vi "IRISS_FPGA_IO_v3.3b.vi"() -> ()   [LabVIEW 2013]
doc: "This VI contains a basic quadrature decoder which is reset asynchronously upon clicking the reset button."
uses:
  <vilib>/Platform/TimedLoop/XDataNode/timing_clust.ctl
  <vilib>/Platform/TimedLoop/XDataNode/nitl_modes.ctl
  <vilib>/Platform/TimedLoop/XDataNode/wakeup.ctl
  <vilib>/rvi/Emulation/niFpgaSctlEmulationGetInTimedLoop.vi
  <vilib>/rvi/Emulation/niFpgaEmulationReportErrorSimple.vi
  <vilib>/rvi/Emulation/niFpgaGetClockAttributes.vi
  <vilib>/rvi/Emulation/niFpgaCriticalErrorInLSC.vi
  <vilib>/rvi/eio/common/nirviEmuTemplateMethod_errors.vi
  <vilib>/platform/TimedLoop/XDataNode/XDataNode.xnode
  <vilib>/eio/EIONode/EIONode.xnode
  <vilib>/Platform/TimedLoop/XDataNode/XDNodeRunTimeDep.lvlib
  Library/KevinLibraryAll/labview/KevLib01.lvlib
  Library/jmslib.lvlib
panel:
  in  "Connector2/DIO10":bool
  in  "Connector2/DIO9":bool
  in  "Connector2/DIO8":bool
  in  "Connector2/DIO7":bool
  in  "Period 1 (Ticks)":u32=1000
  in  "PWM1":fxp<+,32,0>
  in  "Period (Ticks)":u32=2000
  in  "DIR OCT Mot":bool
  in  "INHB OCT Mot":bool
  out "FAULT OCT Mot":bool
  out "Position OCT Mot":i32
  out "JumpBy2Error OCT Mot":i16
  in  "Reset OCT Mot":bool
  in  "OCT Mot DC":fxp<+,32,0>
  in  "Conn0/DIO15 Button 4":bool
  in  "Conn0/DIO12 Button 1":bool
  in  "Conn0/DIO13 Button 2":bool
  out "Home OCT z":bool
  in  "DIR Y":bool
  in  "INHB Y":bool
  out "FAULT Y":bool
  out "Position Y":i32
  out "JumpBy2Error Y":i16
  in  "Reset Y":bool
  in  "Y DC":fxp<+,32,0>
  in  "DIR X":bool
  in  "INHB X":bool
  out "FAULT X":bool
  out "Position X":i32
  out "JumpBy2Error X":i16
  in  "Reset X":bool
  in  "DIR Z":bool
  in  "INHB Z":bool
  out "FAULT Z":bool
  out "Position Z":i32
  out "JumpBy2Error Z":i16
  in  "Reset Z":bool
  in  "Z DC":fxp<+,32,0>
  in  "X DC":fxp<+,32,0>
  out "samples":i32
  out "Current Monitor":u32[](array[numeric])
  out "Raw Data Response (MSB)":bool[](array[boolean])
  out "Home L4":bool
  out "Home L1":bool
  out "Home L2":bool
  out "Home L3":bool
  in  "Positive Direction C1-4":bool
  out "JumpBy2Error C1-4":i16
  out "32 bit Position C1-4":i32
  in  "Reset C1-4":bool
  in  "Positive Direction C1-1":bool
  out "JumpBy2Error C1-1":i16
  out "32 bit Position C1-1":i32
  in  "Reset C1-1":bool
  out "32 bit Position 17":i32
  in  "Reset 17":bool
  in  "Positive Direction 17":bool
  out "JumpBy2Error 17":i16
  out "32 bit Position 16":i32
  in  "Reset 16":bool
  in  "Positive Direction 16":bool
  out "JumpBy2Error 16":i16
  out "32 bit Position 15":i32
  in  "Reset 15":bool
  in  "Positive Direction 15":bool
  out "JumpBy2Error 15":i16
  out "32 bit Position 14":i32
  in  "Reset 14":bool
  in  "Positive Direction 14":bool
  out "JumpBy2Error 14":i16
  out "32 bit Position 13":i32
  in  "Reset 13":bool
  in  "Positive Direction 13":bool
  out "JumpBy2Error 13":i16
  out "32 bit Position 12":i32
  in  "Reset 12":bool
  in  "Positive Direction 12":bool
  out "JumpBy2Error 12":i16
  out "32 bit Position 10":i32
  in  "Reset 10":bool
  in  "Positive Direction 10":bool
  out "JumpBy2Error 10":i16
  out "32 bit Position 9":i32
  in  "Reset 9":bool
  in  "Positive Direction 9":bool
  out "JumpBy2Error 9":i16
  out "JumpBy2Error 3":i16
  in  "Positive Direction 3":bool
  out "JumpBy2Error 1":i16
  in  "Positive Direction 1":bool
  out "AI":i16[](array[numeric])
  out "32 bit Position 3":i32
  in  "Reset 3":bool
  in  "AO":i16[](array[numeric])=[0, 0, 0, 0, 0, 0, 0, 0]
  out "32 bit Position 1":i32
  in  "Reset 1":bool
  # "syringe pump"
  # "Accurus Buttons"
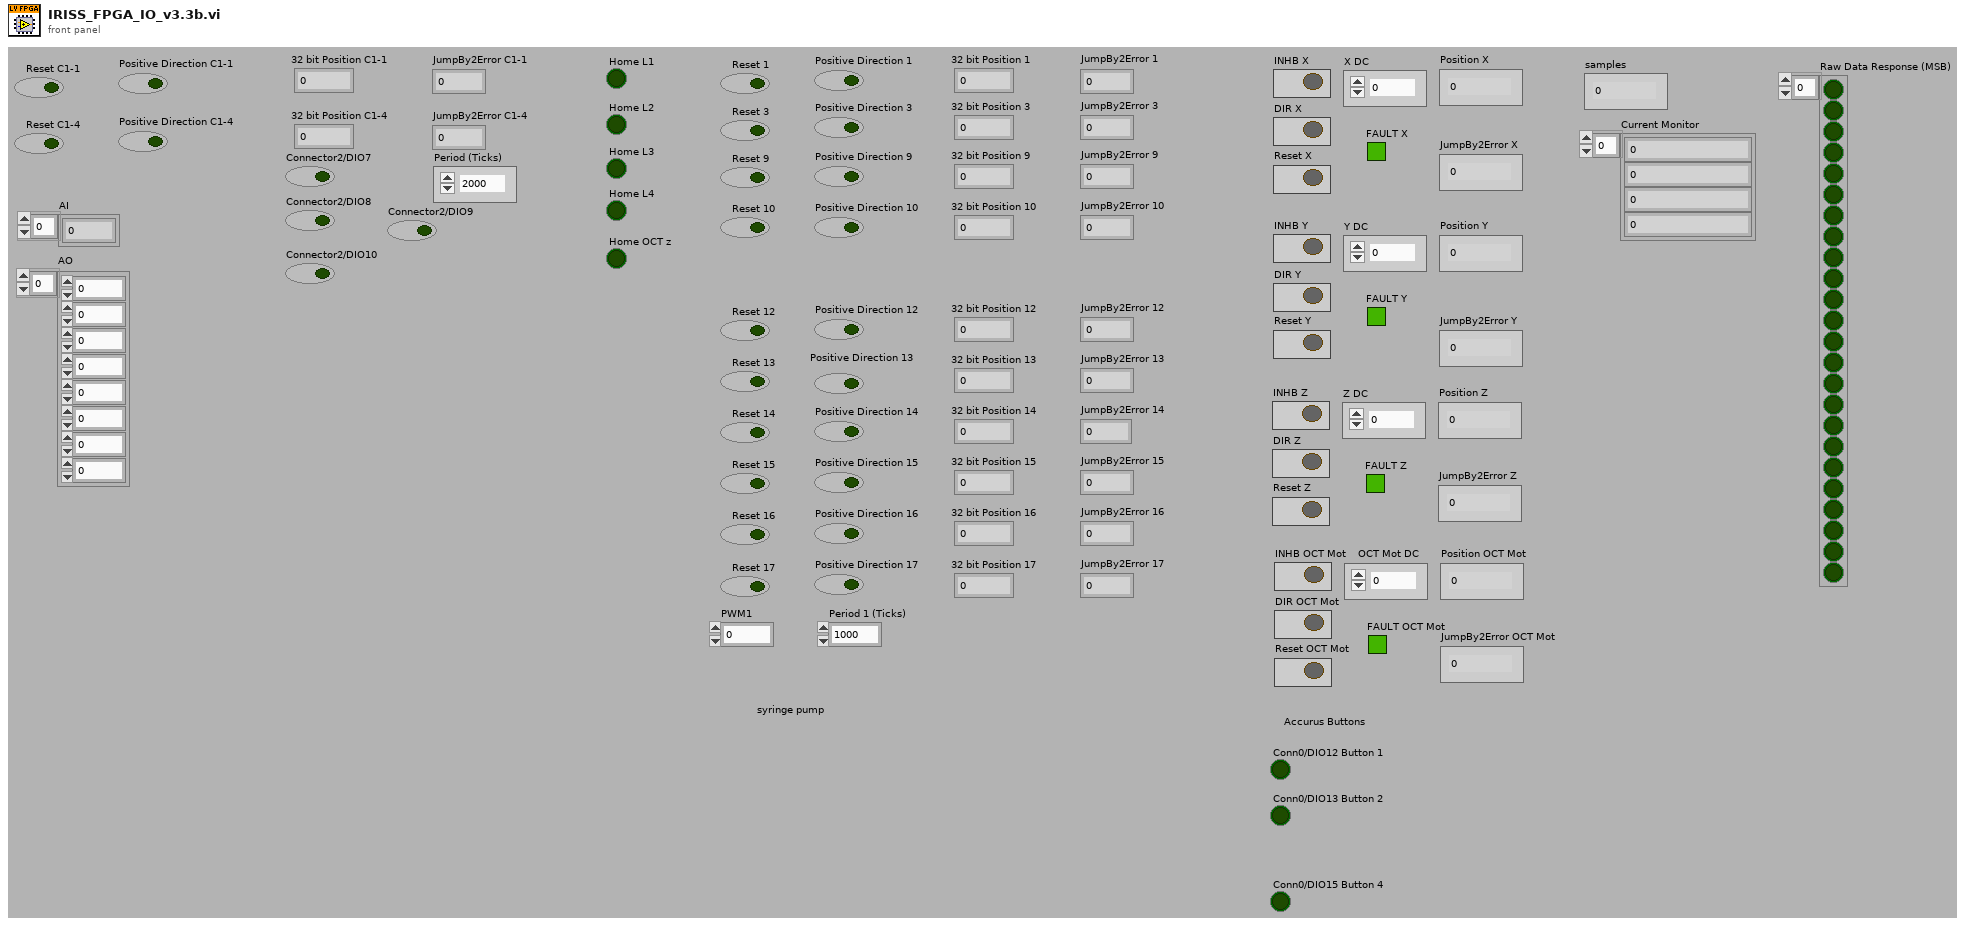
[diagram p1: front panel]
types:
  T1 = typedef "XDNodeRunTimeDep.lvlib/timing_clust.ctl" = cluster{"Expected End [f-1]":u64, "Actual End [f-1]":u64, "Finished Late? [f-1]":bool, "Expected End [i-1]":u64, "Actual End [i-1]":u64, "Finished Late? [i-1]":bool, "Expected Start [i]":u64, "Actual Start [i]":u64, "Expected Start [f]":u64, "Actual Start [f]":u64, "Source Name":string, "Structure Name":string, "Period":i64, "Deadline":i64, "Offset":i64, "Start":i64, "Priority":i32, "Timeout":i32, "Mode":T2, "Wakeup Reason":T3, "Error":errorcluster, "Source Type":string, "Secondary Source Type":string, "Global End Time":u64, "Global Start Time":u64, "Frame Duration":u64, "Iteration Duration":u64, "Assigned CPU":i32, "I/O Scan Engine Mode":u32}
  T2 = typedef "XDNodeRunTimeDep.lvlib/nitl_modes.ctl" = enum32{"No Change", "Process missed periods, maintain original phase", "Discard missed periods, maintain original phase", "Process missed periods, ignore original phase", "Discard missed periods, ignore original phase"}
  T3 = typedef "XDNodeRunTimeDep.lvlib/wakeup.ctl" = enum32{"Normal", "Aborted", "Asynchronous wakeup", "Timing source error", "Timed loop error", "Timeout"}
  T4 = cluster{"PWM In":refnum<k21>, "Direction":refnum<k21>, "Inhibit":refnum<k21>, "Encoder C":refnum<k21>, "Encoder B":refnum<k21>, "Encoder A":refnum<k21>, "Fault":refnum<k21>}
  T5 = cluster{"SCLK":refnum<k21>, "MOSI":refnum<k21>, "MISO":refnum<k21>}
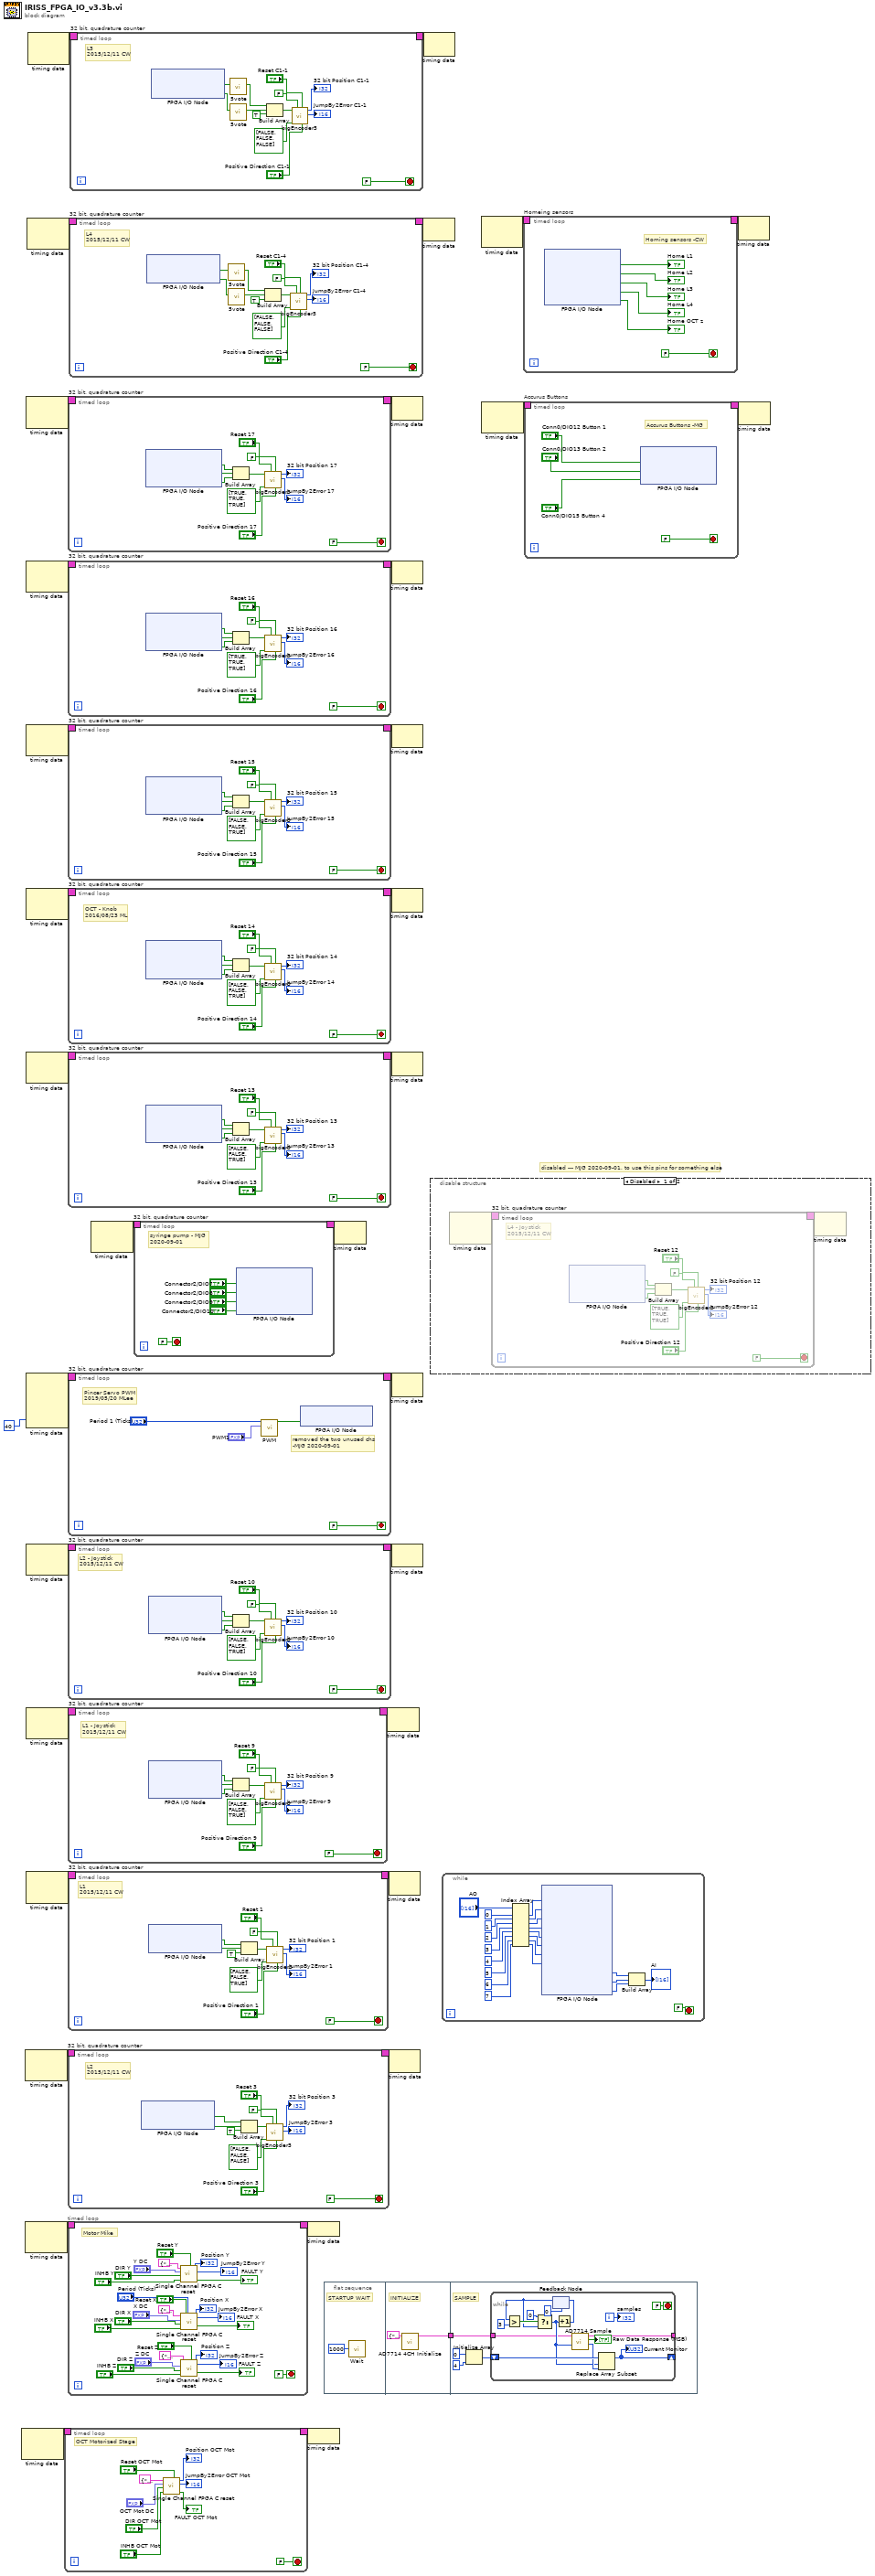
[diagram p0: block diagram]
diagram:
  # "disabled --- MJG 2020-09-01, to use this pins for something else"
  n1 = node-c288() -> (w5:T1)  [unwired: 2 in]
  n2 = node-c288() -> (w34:T1)  [unwired: 2 out]
  n3 = node-c288() -> (w10:T1)  [unwired: 2 in]
  n4 = node-c288() -> (w18:T1)  [unwired: 2 out]
  n5 = node-c288() -> (w20:T1)  [unwired: 2 out]
  n6 = node-c288() -> (w22:T1)  [unwired: 2 out]
  n7 = node-c288() -> (w24:T1)  [unwired: 2 out]
  n8 = node-c288() -> (w26:T1)  [unwired: 2 out]
  n9 = node-c288(i64 40 ("Period")) -> (w28:T1)  [unwired: 3 in, 1 out]
  n10 = node-c288() -> (w30:T1)  [unwired: 2 out]
  n11 = node-c288() -> (w32:T1)  [unwired: 2 out]
  n12 = node-c288() -> (w35:T1)  [unwired: 2 out]
  n13 = node-c288() -> (w14:T1)  [unwired: 2 out]
  n14 = node-c288() -> (w16:T1)  [unwired: 2 out]
  n15 = timed-loop {
    timing: w5 -> [_]
    timing-out: [_] -> w4
    stop <- FALSE stop-if-true
    # "OCT Motorized Stage"
    n16 = call "Single Channel FPGA C reset.vi"("Reset"="Reset OCT Mot", "INHB"="INHB OCT Mot", "DIR"="DIR OCT Mot", "Duty"="OCT Mot DC", "IO Channels"=T4 {"PWM In"="Connector1/DIO7", "Direction"="Connector1/DIO8", "Inhibit"="Connector1/DIO9", "Encoder C"="Connector1/DIO10", "Encoder B"="Connector1/DIO11", "Encoder A"="Connector1/DIO12", "Fault"="Connector1/DIO13"}) -> ("FAULT"=→"FAULT OCT Mot":bool, "JumpBy2Error"=→"JumpBy2Error OCT Mot":i16, "Position"=→"Position OCT Mot":i32)  [unwired: 4 in]
  }
  n17 = timed-loop "32 bit, quadrature counter" {
    timing-out: [_] -> w33
    timing: w34 -> [_]
    stop <- FALSE stop-if-true
    # "L2\n2015/12/11 CW"
    n18 = xnode "FPGA I/O Node"() -> ("Connector0/DIO2"=w51:bool, "Connector0/DIO3"=w50:bool)  [unwired: 2 in, 2 out]
    n19 = Build Array(w51, w50, TRUE ("element")) -> (w57:bool[])
    n20 = call "bigEncoder3.vi"("Positive Direction"="Positive Direction 3", "ForceReset"="Reset 3", "Allow C Reset?"=FALSE, "Reset Array"=bool[] [FALSE, FALSE, FALSE], "Encoder Array"=w57) -> ("JumpBy2Error"=→"JumpBy2Error 3":i16, "Position"=→"32 bit Position 3":i32)  [unwired: 5 out]
  }
  n21 = timed-loop {
    timing: w10 -> [_]
    timing-out: [_] -> w9
    stop <- FALSE stop-if-true
    # "Motor Mike"
    n22 = call "Single Channel FPGA C reset.vi"("Reset"="Reset Y", "INHB"="INHB Y", "DIR"="DIR Y", "Duty"="Y DC", "IO Channels"=T4 {"PWM In"="Connector1/DIO1", "Direction"="Connector1/DIO2", "Inhibit"="Connector1/DIO3", "Encoder C"="Connector1/DIO4", "Encoder B"="Connector1/DIO5", "Encoder A"="Connector1/DIO6", "Fault"="Connector1/DIO0"}) -> ("FAULT"=→"FAULT Y":bool, "JumpBy2Error"=→"JumpBy2Error Y":i16, "Position"=→"Position Y":i32)  [unwired: 4 in]
    n23 = call "Single Channel FPGA C reset.vi"("Reset"="Reset X", "Period (Ticks)"="Period (Ticks)", "INHB"="INHB X", "DIR"="DIR X", "Duty"="X DC", "IO Channels"=T4 {"PWM In"="Connector1/DIO20", "Direction"="Connector1/DIO21", "Inhibit"="Connector1/DIO22", "Encoder C"="Connector1/DIO23", "Encoder B"="Connector1/DIO24", "Encoder A"="Connector1/DIO25", "Fault"="Connector1/DIO27"}) -> ("FAULT"=→"FAULT X":bool, "JumpBy2Error"=→"JumpBy2Error X":i16, "Position"=→"Position X":i32)  [unwired: 3 in]
    n24 = call "Single Channel FPGA C reset.vi"("Reset"="Reset Z", "INHB"="INHB Z", "DIR"="DIR Z", "Duty"="Z DC", "IO Channels"=T4 {"PWM In"="Connector1/DIO14", "Direction"="Connector1/DIO15", "Inhibit"="Connector1/DIO16", "Encoder C"="Connector1/DIO17", "Encoder B"="Connector1/DIO18", "Encoder A"="Connector1/DIO19", "Fault"="Connector1/DIO26"}) -> ("FAULT"=→"FAULT Z":bool, "JumpBy2Error"=→"JumpBy2Error Z":i16, "Position"=→"Position Z":i32)  [unwired: 4 in]
  }
  n25 = timed-loop "32 bit, quadrature counter" {
    timing-out: [_] -> w17
    timing: w18 -> [_]
    stop <- FALSE stop-if-true
    n26 = xnode "FPGA I/O Node"() -> ("Connector2/DIO24"=w98:bool, "Connector2/DIO25"=w97:bool, "Connector2/DIO26"=w89:bool)  [unwired: 3 in, 3 out]
    n27 = Build Array(w98, w97, w89) -> (w96:bool[])
    n28 = call "bigEncoder3.vi"("Positive Direction"="Positive Direction 17", "ForceReset"="Reset 17", "Allow C Reset?"=FALSE, "Reset Array"=bool[] [TRUE, TRUE, TRUE], "Encoder Array"=w96) -> ("JumpBy2Error"=→"JumpBy2Error 17":i16, "Position"=→"32 bit Position 17":i32)  [unwired: 5 out]
  }
  n29 = timed-loop "32 bit, quadrature counter" {
    timing-out: [_] -> w19
    timing: w20 -> [_]
    stop <- FALSE stop-if-true
    n30 = xnode "FPGA I/O Node"() -> ("Connector2/DIO21"=w111:bool, "Connector2/DIO22"=w110:bool, "Connector2/DIO23"=w102:bool)  [unwired: 3 in, 3 out]
    n31 = Build Array(w111, w110, w102) -> (w109:bool[])
    n32 = call "bigEncoder3.vi"("Positive Direction"="Positive Direction 16", "ForceReset"="Reset 16", "Allow C Reset?"=FALSE, "Reset Array"=bool[] [TRUE, TRUE, TRUE], "Encoder Array"=w109) -> ("JumpBy2Error"=→"JumpBy2Error 16":i16, "Position"=→"32 bit Position 16":i32)  [unwired: 5 out]
  }
  n33 = timed-loop "32 bit, quadrature counter" {
    timing-out: [_] -> w21
    timing: w22 -> [_]
    stop <- FALSE stop-if-true
    n34 = xnode "FPGA I/O Node"() -> ("Connector2/DIO18"=w124:bool, "Connector2/DIO19"=w123:bool, "Connector2/DIO20"=w115:bool)  [unwired: 3 in, 3 out]
    n35 = Build Array(w124, w123, w115) -> (w122:bool[])
    n36 = call "bigEncoder3.vi"("Positive Direction"="Positive Direction 15", "ForceReset"="Reset 15", "Allow C Reset?"=FALSE, "Reset Array"=bool[] [FALSE, FALSE, TRUE], "Encoder Array"=w122) -> ("JumpBy2Error"=→"JumpBy2Error 15":i16, "Position"=→"32 bit Position 15":i32)  [unwired: 5 out]
  }
  n37 = timed-loop "32 bit, quadrature counter" {
    timing-out: [_] -> w23
    timing: w24 -> [_]
    stop <- FALSE stop-if-true
    # "OCT - Knob\n2016/08/23 ML"
    n38 = xnode "FPGA I/O Node"() -> ("Connector2/DIO15"=w137:bool, "Connector2/DIO16"=w136:bool, "Connector2/DIO17"=w128:bool)  [unwired: 3 in, 3 out]
    n39 = Build Array(w137, w136, w128) -> (w135:bool[])
    n40 = call "bigEncoder3.vi"("Positive Direction"="Positive Direction 14", "ForceReset"="Reset 14", "Allow C Reset?"=FALSE, "Reset Array"=bool[] [FALSE, FALSE, TRUE], "Encoder Array"=w135) -> ("JumpBy2Error"=→"JumpBy2Error 14":i16, "Position"=→"32 bit Position 14":i32)  [unwired: 5 out]
  }
  n41 = timed-loop "32 bit, quadrature counter" {
    timing-out: [_] -> w25
    timing: w26 -> [_]
    stop <- FALSE stop-if-true
    n42 = xnode "FPGA I/O Node"() -> ("Connector2/DIO12"=w150:bool, "Connector2/DIO13"=w149:bool, "Connector2/DIO14"=w141:bool)  [unwired: 3 in, 3 out]
    n43 = Build Array(w150, w149, w141) -> (w148:bool[])
    n44 = call "bigEncoder3.vi"("Positive Direction"="Positive Direction 13", "ForceReset"="Reset 13", "Allow C Reset?"=FALSE, "Reset Array"=bool[] [FALSE, FALSE, TRUE], "Encoder Array"=w148) -> ("JumpBy2Error"=→"JumpBy2Error 13":i16, "Position"=→"32 bit Position 13":i32)  [unwired: 5 out]
  }
  n45 = timed-loop "32 bit, quadrature counter" {
    timing-out: [_] -> w27
    timing: w28 -> [_]
    stop <- FALSE stop-if-true
    # "removed the two unused chs\n-MJG 2020-09-01"
    # "Pincer Servo PWM\n2019/05/20 MLee"
    n46 = call "PWM.vi"("Duty Cycle"="PWM1", "Period (Ticks)"="Period 1 (Ticks)") -> ("PWM Out"=w156:bool)  [unwired: 8 in, 1 out]
    n47 = xnode "FPGA I/O Node"("Connector2/DIO6"=w156) -> ()  [unwired: 1 in, 1 out]
  }
  n48 = timed-loop "32 bit, quadrature counter" {
    timing-out: [_] -> w29
    timing: w30 -> [_]
    stop <- FALSE stop-if-true
    # "L2 - Joystick\n2015/12/11 CW"
    n49 = xnode "FPGA I/O Node"() -> ("Connector2/DIO3"=w169:bool, "Connector2/DIO4"=w168:bool, "Connector2/DIO5"=w160:bool)  [unwired: 3 in, 3 out]
    n50 = Build Array(w169, w168, w160) -> (w167:bool[])
    n51 = call "bigEncoder3.vi"("Positive Direction"="Positive Direction 10", "ForceReset"="Reset 10", "Allow C Reset?"=FALSE, "Reset Array"=bool[] [FALSE, FALSE, TRUE], "Encoder Array"=w167) -> ("JumpBy2Error"=→"JumpBy2Error 10":i16, "Position"=→"32 bit Position 10":i32)  [unwired: 5 out]
  }
  n52 = timed-loop "32 bit, quadrature counter" {
    timing-out: [_] -> w31
    timing: w32 -> [_]
    stop <- FALSE stop-if-true
    # "L1 - Joystick\n2015/12/11 CW"
    n53 = xnode "FPGA I/O Node"() -> ("Connector2/DIO0"=w182:bool, "Connector2/DIO1"=w181:bool, "Connector2/DIO2"=w173:bool)  [unwired: 3 in, 3 out]
    n54 = Build Array(w182, w181, w173) -> (w180:bool[])
    n55 = call "bigEncoder3.vi"("Positive Direction"="Positive Direction 9", "ForceReset"="Reset 9", "Allow C Reset?"=FALSE, "Reset Array"=bool[] [FALSE, FALSE, TRUE], "Encoder Array"=w180) -> ("JumpBy2Error"=→"JumpBy2Error 9":i16, "Position"=→"32 bit Position 9":i32)  [unwired: 5 out]
  }
  n56 = timed-loop "32 bit, quadrature counter" {
    timing-out: [_] -> w36
    timing: w35 -> [_]
    stop <- FALSE stop-if-true
    # "L1\n2015/12/11 CW"
    n57 = xnode "FPGA I/O Node"() -> ("Connector0/DIO0"=w195:bool, "Connector0/DIO1"=w194:bool)  [unwired: 2 in, 2 out]
    n58 = Build Array(w195, w194, TRUE ("element")) -> (w193:bool[])
    n59 = call "bigEncoder3.vi"("Positive Direction"="Positive Direction 1", "ForceReset"="Reset 1", "Allow C Reset?"=FALSE, "Reset Array"=bool[] [FALSE, FALSE, TRUE], "Encoder Array"=w193) -> ("JumpBy2Error"=→"JumpBy2Error 1":i16, "Position"=→"32 bit Position 1":i32)  [unwired: 5 out]
  }
  n60 = timed-loop "32 bit, quadrature counter" {
    timing-out: [_] -> w13
    timing: w14 -> [_]
    stop <- FALSE stop-if-true
    # "L4\n2015/12/11 CW"
    n61 = xnode "FPGA I/O Node"() -> ("Connector0/DIO6"=w202:bool, "Connector0/DIO7"=w201:bool)  [unwired: 2 in, 2 out]
    n62 = call "5vote.vi"("Input"=w202) -> ("vote5"=w199:bool)  [unwired: 10 in]
    n63 = call "5vote.vi"("Input"=w201) -> ("vote5"=w200:bool)  [unwired: 10 in]
    n64 = Build Array(w199, w200, TRUE ("element")) -> (w210:bool[])
    n65 = call "bigEncoder3.vi"("Positive Direction"="Positive Direction C1-4", "ForceReset"="Reset C1-4", "Allow C Reset?"=FALSE, "Reset Array"=bool[] [FALSE, FALSE, FALSE], "Encoder Array"=w210) -> ("JumpBy2Error"=→"JumpBy2Error C1-4":i16, "Position"=→"32 bit Position C1-4":i32)  [unwired: 5 out]
  }
  n66 = timed-loop "32 bit, quadrature counter" {
    timing-out: [_] -> w15
    timing: w16 -> [_]
    stop <- FALSE stop-if-true
    # "L3\n2015/12/11 CW"
    n67 = xnode "FPGA I/O Node"() -> ("Connector0/DIO4"=w217:bool, "Connector0/DIO5"=w216:bool)  [unwired: 2 in, 2 out]
    n68 = call "5vote.vi"("Input"=w217) -> ("vote5"=w214:bool)  [unwired: 10 in]
    n69 = call "5vote.vi"("Input"=w216) -> ("vote5"=w215:bool)  [unwired: 10 in]
    n70 = Build Array(w214, w215, TRUE ("element")) -> (w225:bool[])
    n71 = call "bigEncoder3.vi"("Positive Direction"="Positive Direction C1-1", "ForceReset"="Reset C1-1", "Allow C Reset?"=FALSE, "Reset Array"=bool[] [FALSE, FALSE, FALSE], "Encoder Array"=w225) -> ("JumpBy2Error"=→"JumpBy2Error C1-1":i16, "Position"=→"32 bit Position C1-1":i32)  [unwired: 5 out]
  }
  n72 = node-c288() -> (w2:T1)  [unwired: 2 out]
  n73 = timed-loop "32 bit, quadrature counter" {
    timing-out: [_] -> w1
    timing: w2 -> [_]
    stop <- FALSE stop-if-true
    # "syringe pump - MJG \n2020-09-01"
    n74 = xnode "FPGA I/O Node"("Connector2/DIO7"="Connector2/DIO7", "Connector2/DIO8"="Connector2/DIO8", "Connector2/DIO9"="Connector2/DIO9", "Connector2/DIO10"="Connector2/DIO10") -> ()  [unwired: 4 in, 4 out]
  }
  n75 = node-c288(w9) -> ()
  n76 = node-c288(w4) -> ()
  n77 = flat-sequence {
    tunnel: [w237] -> w8
    tunnel: w8 -> [w239]
    frame #0 {
      # "STARTUP WAIT"
      n78 = call "Wait"("Count(uSec)"=u32 1000) -> ()  [unwired: 1 out]
    }
    frame #1 {
      # "INITIALIZE"
      n79 = call "AD7714 4CH Initialize.vi"("I/O Cluster In"=T5 {"SCLK"="Connector1/DIO29", "MOSI"="Connector1/DIO35", "MISO"="Connector1/DIO31"}) -> ("I/O Cluster Out"=w237:T5)  [unwired: 10 in]
    }
    frame #2 {
      # "SAMPLE"
      n80 = Initialize Array(u32 0, 4 ("dimension size")) -> (w240:u32[])
      n81 = while {
        shift-right: [w248] -> _
        shift-left: w240 -> [w249]
        tunnel: w239 -> [w245]
        tunnel: [w244] -> _
        i -> [w256]
        stop <- FALSE stop-if-true
        n82 = feedback #1(i16 0) -> (w252:i16)
        n83 = Greater?(x=w252, y=i16 3) -> (0:w253:bool)
        n84 = Select(t=i16 0, s=w253, f=w252) -> (s? t:f=w246:i16)
        n85 = Increment(x=w246) -> (x+1=w250:i16)
        n86 = feedback-in #1(w250) -> ()
        n87 = call "AD7714 Sample.vi"("Channel"=w246, "I/O Cluster In"=w245) -> ("Data"=w247:u32, "Raw Data Response (MSB)"=→"Raw Data Response (MSB)":bool[], "I/O Cluster Out"=w244:T5)  [unwired: 7 in]
        n88 = Replace Array Subset(array=w249, new element=w247, index=w246) -> (w248:u32[])
        "Current Monitor" <- w248
        "samples" <- w256
      }
    }
  }
  n89 = node-c288(w1) -> ()  [unwired: 1 out]
  n90 = node-c288(w31) -> ()  [unwired: 1 out]
  n91 = node-c288(w36) -> ()  [unwired: 1 out]
  n92 = node-c288(w33) -> ()  [unwired: 1 out]
  n93 = node-c288(w17) -> ()  [unwired: 1 out]
  n94 = node-c288(w19) -> ()  [unwired: 1 out]
  n95 = node-c288(w21) -> ()  [unwired: 1 out]
  n96 = node-c288(w23) -> ()  [unwired: 1 out]
  n97 = node-c288(w25) -> ()  [unwired: 1 out]
  n98 = node-c288(w27) -> ()  [unwired: 1 out]
  n99 = node-c288(w29) -> ()  [unwired: 1 out]
  n100 = node-c288(w13) -> ()  [unwired: 1 out]
  n101 = node-c288(w15) -> ()  [unwired: 1 out]
  n102 = disable-structure shown="Disabled" {
    frame Disabled {
      n103 = node-c288() -> (w259:T1)  [unwired: 2 out]
      n104 = timed-loop "32 bit, quadrature counter" {
        timing-out: [_] -> w258
        timing: w259 -> [_]
        stop <- FALSE stop-if-true
        # "L4 - Joystick\n2015/12/11 CW"
        n105 = xnode "FPGA I/O Node"() -> ("Connector2/DIO9"=w269:bool, "Connector2/DIO10"=w268:bool, "Connector2/DIO11"=w260:bool)  [unwired: 3 in, 3 out]
        n106 = Build Array(w269, w268, w260) -> (w267:bool[])
        n107 = call "bigEncoder3.vi"("Positive Direction"="Positive Direction 12", "ForceReset"="Reset 12", "Allow C Reset?"=FALSE, "Reset Array"=bool[] [TRUE, TRUE, TRUE], "Encoder Array"=w267) -> ("JumpBy2Error"=→"JumpBy2Error 12":i16, "Position"=→"32 bit Position 12":i32)  [unwired: 5 out]
      }
      n108 = node-c288(w258) -> ()  [unwired: 1 out]
    }
    frame Enabled {
    }
  }
  n109 = while {
    stop <- FALSE stop-if-true
    n110 = Index Array(array="AO", index #1=0 ("index"), index #2=1 ("index"), index #3=2 ("index"), index #4=3 ("index"), index #5=4 ("index"), index #6=5 ("index"), index #7=6 ("index"), index #8=7 ("index")) -> (element #1=w287:i16, element #2=w286:i16, element #3=w285:i16, element #4=w284:i16, element #5=w283:i16, element #6=w282:i16, element #7=w281:i16, element #8=w280:i16)
    n111 = xnode "FPGA I/O Node"("Connector0/AO0"=w287, "Connector0/AO1"=w286, "Connector0/AO2"=w285, "Connector0/AO3"=w284, "Connector0/AO4"=w283, "Connector0/AO5"=w282, "Connector0/AO6"=w281, "Connector0/AO7"=w280) -> ("Connector0/AI0"=w278:i16, "Connector0/AI1"=w277:i16, "Connector0/AI2"=w275:i16)  [unwired: 11 in, 11 out]
    n112 = Build Array(w278, w277, w275) -> (→"AI":i16[])
  }
  n113 = node-c288() -> (w12:T1)  [unwired: 2 out]
  n114 = node-c288() -> (w7:T1)  [unwired: 2 out]
  n115 = timed-loop "Homeing sensors" {
    timing-out: [_] -> w11
    timing: w12 -> [_]
    stop <- FALSE stop-if-true
    # "Homing sensors -CW"
    n116 = xnode "FPGA I/O Node"() -> ("Connector0/DIO8"=→"Home L1":bool, "Connector0/DIO9"=→"Home L2":bool, "Connector0/DIO10"=→"Home L3":bool, "Connector0/DIO11"=→"Home L4":bool, "Connector0/DIO14"=→"Home OCT z":bool)  [unwired: 5 in, 5 out]
  }
  n117 = timed-loop "Accurus Buttons" {
    timing-out: [_] -> w6
    timing: w7 -> [_]
    stop <- FALSE stop-if-true
    # "Accurus Buttons -MG"
    n118 = xnode "FPGA I/O Node"("Connector0/DIO12"="Conn0/DIO12 Button 1", "Connector0/DIO13"="Conn0/DIO13 Button 2", "Connector0/DIO15"="Conn0/DIO15 Button 4") -> ()  [unwired: 3 in, 3 out]
  }
  n119 = node-c288(w11) -> ()  [unwired: 1 out]
  n120 = node-c288(w6) -> ()  [unwired: 1 out]
